vi "LOER_BuildMenu.vi"(0 "XRef":T8, 1 "MenuRef":T7, 2 "Point":T5, 3 "Menu Type":T4, 4 "State In":T2={"Inputs"=1, "SelectedIndex"=0, "ClassInfo"=[], "Width"=100, "EventReg Type"=variant}) -> (14 "Fatal Error Out":T1)   [LabVIEW 2016, in "LV Object Event Registration Node.xnode"]
uses:
  LV Object Event Registration Node.xnode
  <vilib>/XNodeSupport/XNodeXNodeRef.ctl
  <vilib>/XNodeSupport/XNodeMenuRef.ctl
  <vilib>/XNodeSupport/XNodePoint.ctl
  <vilib>/XNodeSupport/XNodeInt.ctl
  <vilib>/XNodeSupport/XNodeMenuType.ctl
  LOER_State.ctl
  LOER_ClassInfo.ctl
  <vilib>/XNodeSupport/XNodeErrorCluster.ctl
  <vilib>/XNodeSupport/NI_XNodeSupport.lvlib
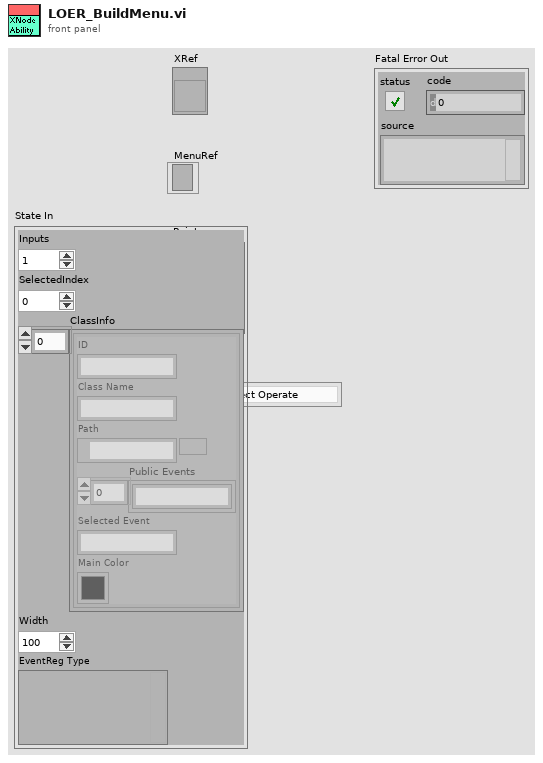
[diagram p1: front panel]
types:
  T1 = typedef "NI_XNodeSupport.lvlib/XNodeErrorCluster.ctl" = errorcluster
  T2 = typedef "LV Object Event Registration Node.xnode/LOER_State.ctl" = cluster{"Inputs":u16, "SelectedIndex":i16, "ClassInfo":T3[], "Width":u16, "EventReg Type":variant}
  T3 = typedef "LV Object Event Registration Node.xnode/LOER_ClassInfo.ctl" = cluster{"ID":string, "Class Name":string, "Path":path, "Public Events":string[], "Selected Event":string, "Main Color":u32}
  T4 = typedef "NI_XNodeSupport.lvlib/XNodeMenuType.ctl" = enum32{"Single Object Operate", "Single Object Popup", "Multi Object Popup Master", "Multi Object Popup Other"}
  T5 = typedef "NI_XNodeSupport.lvlib/XNodePoint.ctl" = cluster{"H":T6, "V":T6}
  T6 = typedef "NI_XNodeSupport.lvlib/XNodeInt.ctl" = i32
  T7 = typedef "NI_XNodeSupport.lvlib/XNodeMenuRef.ctl" = refnum<k9>
  T8 = typedef "NI_XNodeSupport.lvlib/XNodeXNodeRef.ctl" = refnum<vi>
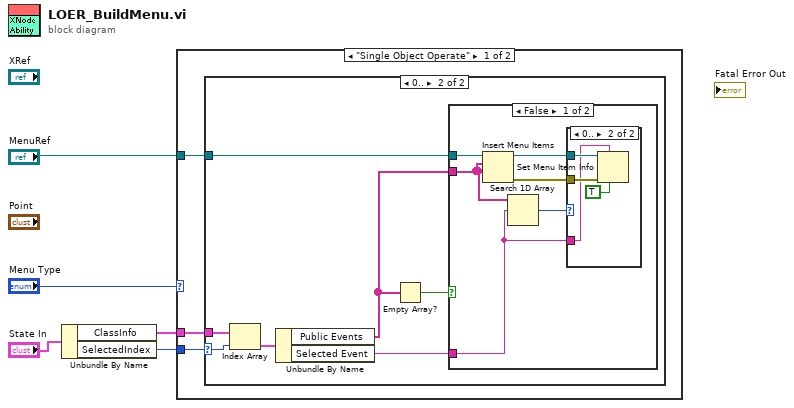
[diagram p0: block diagram]
diagram:
  n1 = Unbundle By Name("State In") -> ("ClassInfo"=w1:T3[], "SelectedIndex"=w3:i16)
  n2 = case shown="\"Single Object Operate\"" "Menu Type" {
    tunnel: w3 -> [w8 _]
    tunnel: "MenuRef" -> [w7 _]
    tunnel: w1 -> [w6 _]
    frame "Single Object Operate" {
      n3 = case shown="0.." w8 {
        selector: w8 -> [_ w13]
        tunnel: w7 -> [_ w15]
        tunnel: w6 -> [_ w14]
        frame Default {
        }
        frame 0.. {
          n4 = Index Array(array=w14, index=w13) -> (element=w12:T3)
          n5 = Unbundle By Name(w12) -> ("Public Events"=w10:string[], "Selected Event"=w9:string)
          n6 = Empty Array?(array=w10) -> (empty?=w11:bool)
          n7 = case shown="False" w11 {
            tunnel: w15 -> [w21 _]
            tunnel: w10 -> [w19 _]
            tunnel: w9 -> [w16 _]
            frame False {
              n8 = Insert Menu Items(7:w19, 8:w19, 9:w21) -> (0:w18:errorcluster, 3:w20:refnum<k9>)  [unwired: 3 in, 1 out]
              n9 = Search 1D Array(1D array=w19, element=w16) -> (index of element=w17:i32)  [unwired: 1 in]
              n10 = case shown="0.." w17 {
                tunnel: w20 -> [_ w25]
                tunnel: w18 -> [_ w24]
                tunnel: w16 -> [_ w22]
                frame Default {
                }
                frame 0.. {
                  n11 = Set Menu Item Info(6:TRUE ("checked"), 7:w22, 8:w24, 11:w25) -> ()  [unwired: 3 in, 2 out]
                }
              }
            }
            frame True {
            }
          }
        }
      }
    }
    frame "Single Object Popup", Default {
    }
  }
